vi "Example2.vi"() -> ()   [LabVIEW 2019]
uses:
  System.Windows.Forms
  source code/MDI Library/Typedef/Tile Direction.ctl
  source code/MDI Library/Typedef/Cascade Order.ctl
  source code/Container/dotNET Container/dotNET Container.lvclass
  D:/Namratha/MDI/LabVIEW-MDI-develop_LV2019/source code/Container/Container base/Container base.lvclass
  source code/Document/LV Doc/Child/LV DEV/LV DEV.lvclass
  D:/Namratha/MDI/LabVIEW-MDI-develop_LV2019/source code/Document/Document base/Document.lvclass
  source code/MDI Library/Public/Create.vi
  source code/Document/LV Doc/Child/LV DEV/public/LV Dev Doc - Instantiate with Path.vi
  source code/Document/LV Doc/Child/LV DEV/public/LV Dev Doc - Instantiate with Ref.vi
  source code/MDI Library/Public/Add.vi
  source code/MDI Library/Public/Show.vi
  source code/MDI Library/Public/Dock.vi
  source code/MDI Library/Public/Tile.vi
  source code/MDI Library/Public/Cascade.vi
  source code/MDI Library/Public/Set Position.vi
  source code/MDI Library/Public/Save.vi
  source code/MDI Library/Public/Remove.vi
  source code/Document/Document base/Document.lvclass
  source code/MDI Library/LV MDI.lvclass
  source code/Document/LV Doc/Child/LV RT/LV RT.lvclass
  source code/Document/LV Doc/Child/LV RT/public/LV RT Doc - Instantiate with Ref.vi
  source code/Document/LV Doc/Child/LV RT/public/LV RT Doc - Instantiate with Path.vi
  D:/Namratha/MDI/LabVIEW-MDI-develop_LV2019/source code/Document/LV Doc/LV Doc.lvclass
panel:
  in  "LV Doc Path":path
  in  "XML File Path":path
  in  "Panel Reference":refnum<k24>(container)
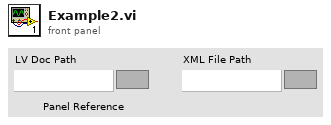
[diagram p1: front panel]
types:
  T1 = typedef "LV MDI.lvclass/Cascade Order.ctl" = u16
  T2 = typedef "LV MDI.lvclass/Tile Direction.ctl" = u16
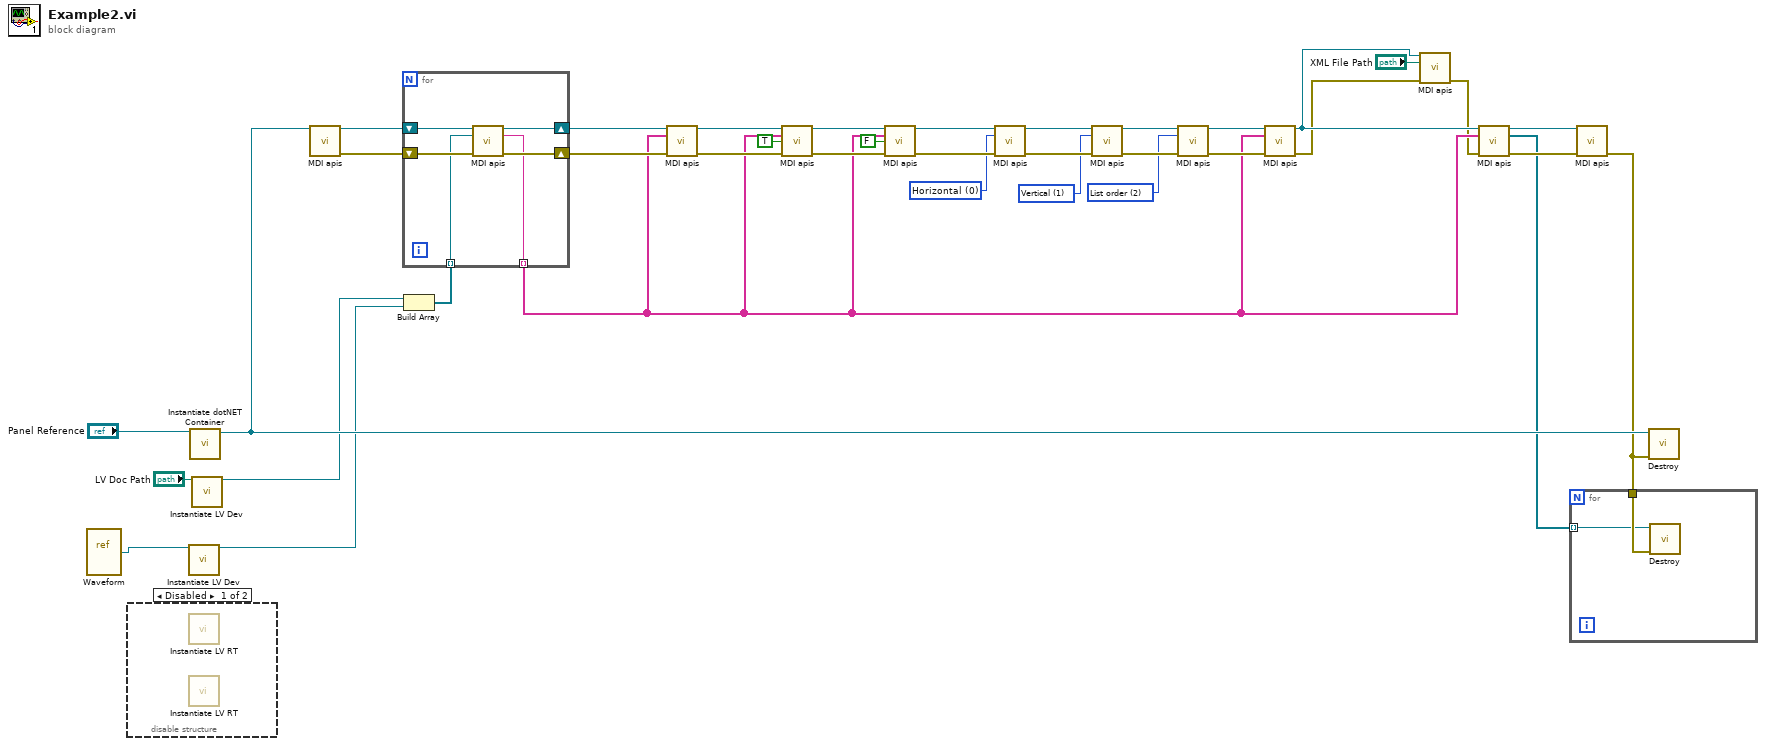
[diagram p0: block diagram]
diagram:
  w6 = T1 2 items=["List order"=2, "Z order"=4] ("Order")
  w7 = T2 1 items=["Horizontal", "Vertical"] ("Tile Direction")
  w8 = T2 0 items=["Horizontal", "Vertical"] ("Tile Direction")
  n1 = vi-ref "Waveform.vi"() -> (w1:refnum<vi>)
  n2 = disable-structure shown="Disabled" {
    frame Disabled {
      n3 = call-poly "Instantiate LV RT.vi"() -> ()  [unwired: 14 in, 2 out]
      n4 = call-poly "Instantiate LV RT.vi"() -> ()  [unwired: 14 in, 2 out]
    }
    frame Enabled {
    }
  }
  n5 = call-poly "Instantiate LV Dev.vi"("VI Refnum"=w1) -> ("LV DEV"=w9:refnum<class "LV DEV.lvclass">)  [unwired: 13 in, 1 out]
  n6 = call "Instantiate dotNET Container.vi"("Panel Reference"="Panel Reference") -> ("dotNET Container out"=w37:refnum<class "dotNET Container.lvclass">)  [unwired: 9 in, 1 out]
  n7 = call-poly "Instantiate LV Dev.vi"("LV Doc Path"="LV Doc Path") -> ("LV DEV"=w10:refnum<class "LV DEV.lvclass">)  [unwired: 13 in, 1 out]
  n8 = call-poly "MDI apis.vi"("Container"=w37) -> ("LV MDI"=w36:refnum<class "LV MDI.lvclass">, "error out"=w35:errorcluster)  [unwired: 13 in]
  n9 = Build Array(w10, w9) -> (w34:refnum<class "LV DEV.lvclass">[])
  n10 = for {
    shift-right: [w41] -> w28
    shift-left: w36 -> [w43]
    shift-right: [w40] -> w27
    shift-left: w35 -> [w42]
    tunnel: w34 -> [w39] mode=indexing
    tunnel: [w38] -> w12 mode=indexing
    n11 = call-poly "MDI apis.vi"("LV MDI.lvclass"=w43, "Document class"=w39, "error in (no error)"=w42) -> ("LV MDI.lvclass"=w41:refnum<class "LV MDI.lvclass">, "Doc UID"=w38:string, "error out"=w40:errorcluster)  [unwired: 10 in]
  }
  n12 = call-poly "MDI apis.vi"("LV MDI in"=w28, "Doc UID[]"=w12, "error in (no error)"=w27) -> ("LV MDI out"=w26:refnum<class "LV MDI.lvclass">, "error out"=w25:errorcluster)  [unwired: 11 in]
  n13 = call-poly "MDI apis.vi"("LV MDI.lvclass"=w26, "Doc UID[]"=w12, "Undock?"=TRUE, "error in (no error)"=w25) -> ("LV MDI.lvclass"=w23:refnum<class "LV MDI.lvclass">, "error out"=w22:errorcluster)  [unwired: 10 in]
  n14 = call-poly "MDI apis.vi"("LV MDI.lvclass"=w23, "Doc UID[]"=w12, "Undock?"=FALSE, "error in (no error)"=w22) -> ("LV MDI.lvclass"=w20:refnum<class "LV MDI.lvclass">, "error out"=w19:errorcluster)  [unwired: 10 in]
  n15 = call-poly "MDI apis.vi"("LV MDI.lvclass"=w20, "Tile Direction"=w8, "error in (no error)"=w19) -> ("LV MDI.lvclass"=w18:refnum<class "LV MDI.lvclass">, "error out"=w17:errorcluster)  [unwired: 11 in]
  n16 = call-poly "MDI apis.vi"("LV MDI.lvclass"=w18, "Tile Direction"=w7, "error in (no error)"=w17) -> ("LV MDI.lvclass"=w16:refnum<class "LV MDI.lvclass">, "error out"=w15:errorcluster)  [unwired: 11 in]
  n17 = call-poly "MDI apis.vi"("LV MDI in"=w16, "Order"=w6, "error in (no error)"=w15) -> ("LV MDI out"=w14:refnum<class "LV MDI.lvclass">, "error out"=w13:errorcluster)  [unwired: 11 in]
  n18 = call-poly "MDI apis.vi"("LV MDI.lvclass"=w14, "Doc UID[]"=w12, "error in (no error)"=w13) -> ("LV MDI.lvclass"=w11:refnum<class "LV MDI.lvclass">, "error out"=w3:errorcluster)  [unwired: 11 in]
  n19 = call-poly "MDI apis.vi"("LV MDI in"=w11, "XML File Path"="XML File Path", "error in (no error)"=w3) -> ("error out"=w2:errorcluster)  [unwired: 11 in, 1 out]
  n20 = call-poly "MDI apis.vi"("LV MDI in"=w11, "Doc UID[]"=w12, "error in (no error)"=w2) -> ("LV MDI out"=w31:refnum<class "LV MDI.lvclass">, "Doc obj[]"=w29:refnum<class "Document.lvclass">[], "error out"=w30:errorcluster)  [unwired: 10 in]
  n21 = call-poly "MDI apis.vi"("LV MDI in"=w31, "error in (no error)"=w30) -> ("error out"=w33:errorcluster)  [unwired: 12 in, 1 out]
  n22 = for {
    tunnel: w33 -> [w45]
    tunnel: w29 -> [w44] mode=indexing
    n23 = call-dynamic "Destroy.vi"("error in (no error)"=w45, "Document in"=w44) -> ()  [unwired: 8 in, 2 out]
  }
  n24 = call-dynamic "Destroy.vi"("error in (no error)"=w33, "dotNET Container in"=w37) -> ()  [unwired: 8 in, 2 out]
